vi "PC104_interface_GUI.vi"(8 "error in (no error)":errorcluster, 9 "URL prefex":string, 10 "Http session":T1, 11 "go":bool=TRUE) -> (2 "error out":errorcluster, 3 "Cluster":T2)   [LabVIEW 2017]
uses:
  Type_Defs/Digital_Out.ctl
  Type_Defs/Digital_In_1.ctl
  Type_Defs/Digital_In_SW_Wire_Faults.ctl
  Type_Defs/Digital_In_SW_States.ctl
  <vilib>/httpClient/ClientHandle.ctl
  msg7171_linux.llb/send single message.vi
  msg7171_linux.llb/send multiple messages.vi
  <vilib>/httpClient/POSTBuffer.vi
  <vilib>/httpClient/LabVIEWHTTPClient.lvlib
panel:
  out "Digi_In_SW_status":T3
  out "Digi_In_SW: Wire Faults":T4
  out "GetAIO json":string
  out "GetDIO json":string
  in  "Get AIO":bool=TRUE
  in  "IR Lamps DutyCycle":dbl[][](array[numeric]) format="%#.4g"
  in  "LN2 Platen":u16(slide) max=2047 step=1 scale=0.0..2047.0
  in  "LN2 Shroud":u16(slide) max=2047 step=1 scale=0.0..2047.0
  out "Digi_In_Bits":T5
  in  "Digi_Out":T6
  in  "Get DIO":bool=TRUE
  in  "exit":bool
  # "1"
  # "15"
  # "2"
  # "16"
  # "2              4              6              8              10            12            14          16"
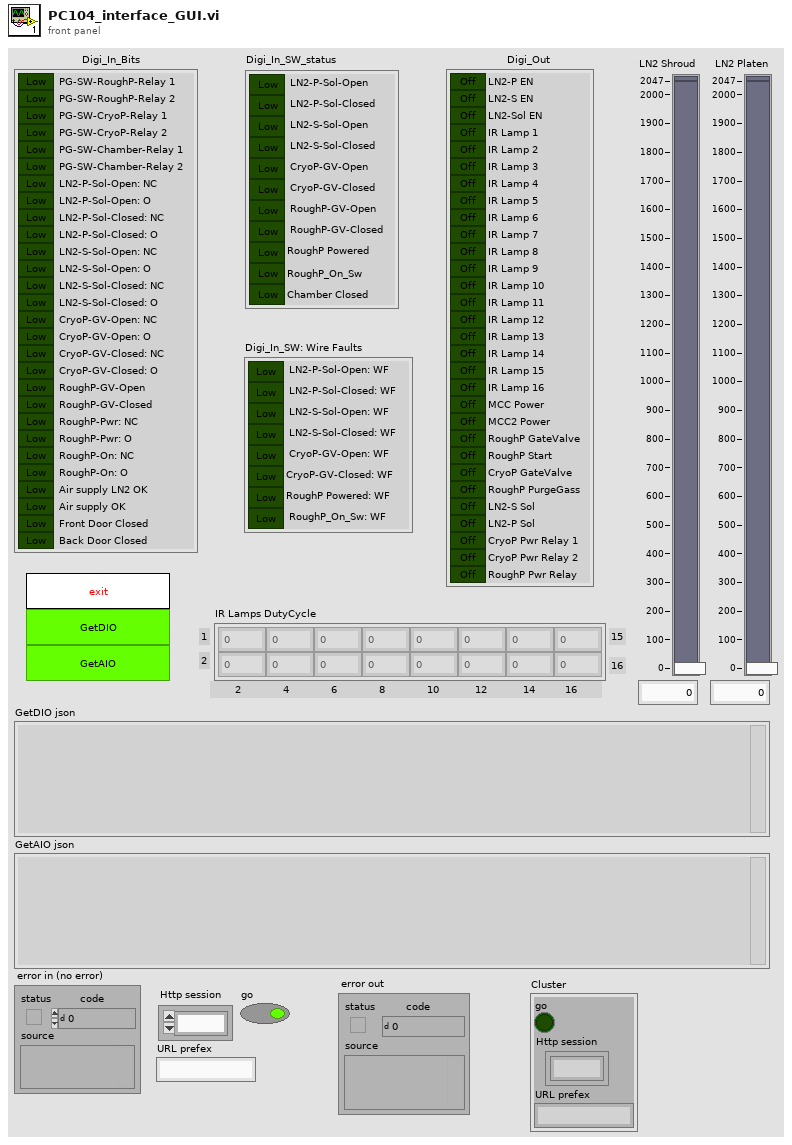
[diagram p1: front panel]
types:
  T1 = typedef "LabVIEWHTTPClient.lvlib/ClientHandle.ctl" = refnum<k1>
  T2 = cluster{"go":bool, "Http session":T1, "URL prefex":string}
  T3 = typedef "Digital_In_SW_States.ctl" = cluster{"LN2-P-Sol-Open":bool, "LN2-P-Sol-Closed":bool, "LN2-S-Sol-Open":bool, "LN2-S-Sol-Closed":bool, "CryoP-GV-Open":bool, "CryoP-GV-Closed":bool, "RoughP-GV-Open":bool, "RoughP-GV-Closed":bool, "RoughP Powered":bool, "RoughP_On_Sw":bool, "Chamber Closed":bool}
  T4 = typedef "Digital_In_SW_Wire_Faults.ctl" = cluster{"LN2-P-Sol-Open: WF":bool, "LN2-P-Sol-Closed: WF":bool, "LN2-S-Sol-Open: WF":bool, "LN2-S-Sol-Closed: WF":bool, "CryoP-GV-Open: WF":bool, "CryoP-GV-Closed: WF":bool, "RoughP Powered: WF":bool, "RoughP_On_Sw: WF":bool}
  T5 = typedef "Digital_In_1.ctl" = cluster{"PG-SW-RoughP-Relay 1":bool, "PG-SW-RoughP-Relay 2":bool, "PG-SW-CryoP-Relay 1":bool, "PG-SW-CryoP-Relay 2":bool, "PG-SW-Chamber-Relay 1":bool, "PG-SW-Chamber-Relay 2":bool, "LN2-P-Sol-Open: NC":bool, "LN2-P-Sol-Open: O":bool, "LN2-P-Sol-Closed: NC":bool, "LN2-P-Sol-Closed: O":bool, "LN2-S-Sol-Open: NC":bool, "LN2-S-Sol-Open: O":bool, "LN2-S-Sol-Closed: NC":bool, "LN2-S-Sol-Closed: O":bool, "CryoP-GV-Open: NC":bool, "CryoP-GV-Open: O":bool, "CryoP-GV-Closed: NC":bool, "CryoP-GV-Closed: O":bool, "RoughP-GV-Open":bool, "RoughP-GV-Closed":bool, "RoughP-Pwr: NC":bool, "RoughP-Pwr: O":bool, "RoughP-On: NC":bool, "RoughP-On: O":bool, "Air supply LN2 OK":bool, "Air supply OK":bool, "Front Door Closed":bool, "Back Door Closed":bool}
  T6 = typedef "Digital_Out.ctl" = cluster{"LN2-P EN":bool, "LN2-S EN":bool, "LN2-Sol EN":bool, "IR Lamp 1":bool, "IR Lamp 2":bool, "IR Lamp 3":bool, "IR Lamp 4":bool, "IR Lamp 5":bool, "IR Lamp 6":bool, "IR Lamp 7":bool, "IR Lamp 8":bool, "IR Lamp 9":bool, "IR Lamp 10":bool, "IR Lamp 11":bool, "IR Lamp 12":bool, "IR Lamp 13":bool, "IR Lamp 14":bool, "IR Lamp 15":bool, "IR Lamp 16":bool, "MCC Power":bool, "MCC2 Power":bool, "RoughP GateValve":bool, "RoughP Start":bool, "CryoP GateValve":bool, "RoughP PurgeGass":bool, "LN2-S Sol":bool, "LN2-P Sol":bool, "CryoP Pwr Relay 1":bool, "CryoP Pwr Relay 2":bool, "RoughP Pwr Relay":bool}
  T7 = cluster{"out":T6, "in bits":T5, "in sw":T3, "sw wf":T4}
  T8 = cluster{"out":cluster{"LN2 Platen":u16, "LN2 Shroud":u16}}
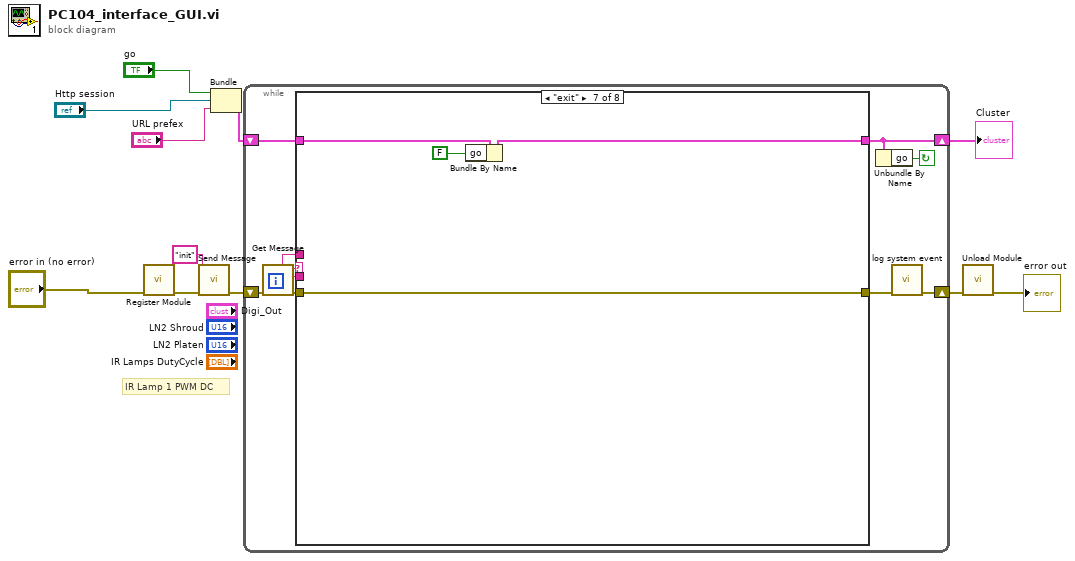
[diagram p0: block diagram]
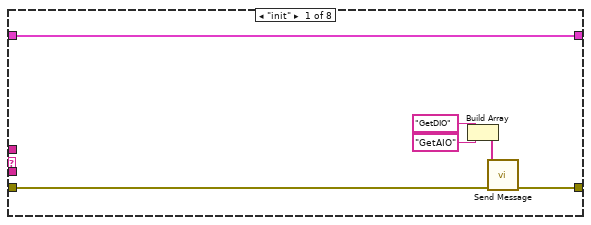
[diagram p2: hidden frame]
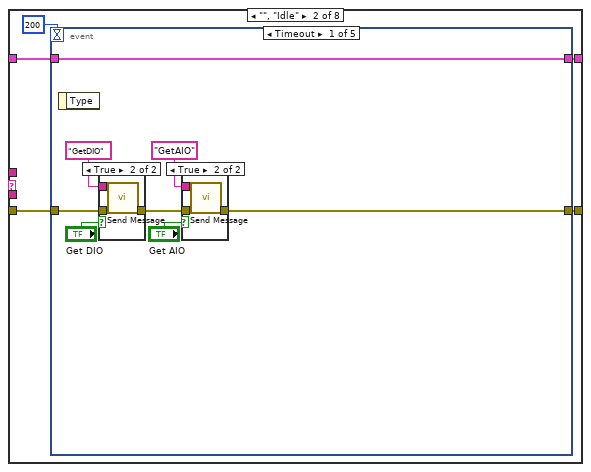
[diagram p3: hidden frame]
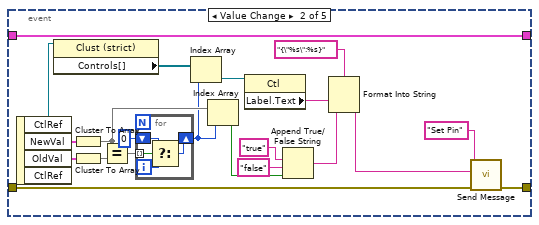
[diagram p6: hidden frame]
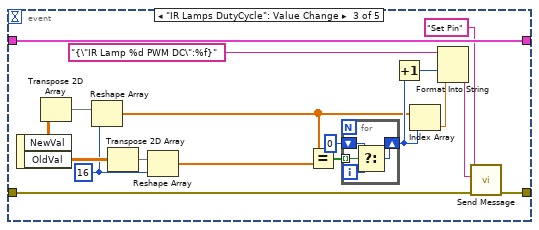
[diagram p7: hidden frame]
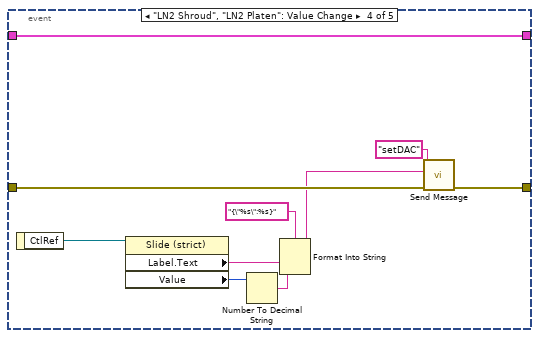
[diagram p8: hidden frame]
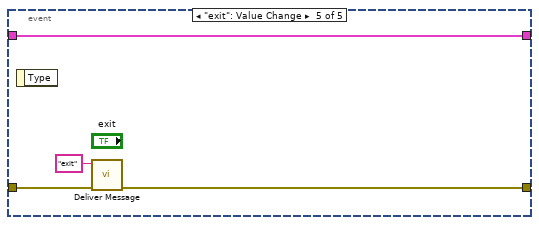
[diagram p9: hidden frame]
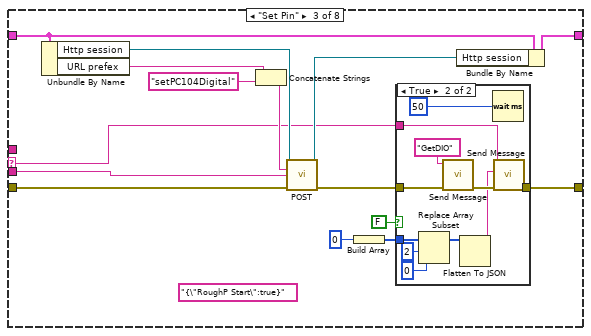
[diagram p10: hidden frame]
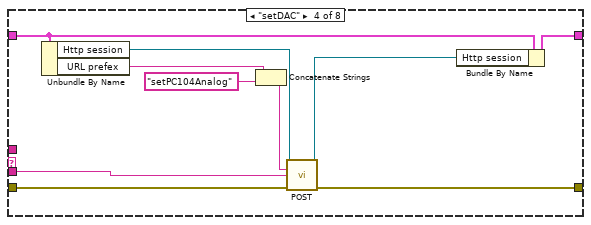
[diagram p12: hidden frame]
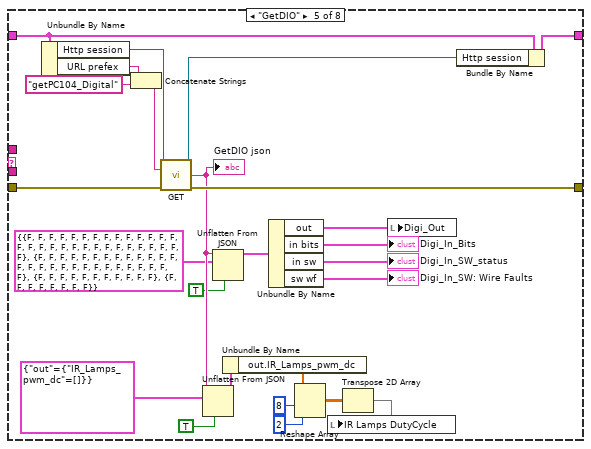
[diagram p13: hidden frame]
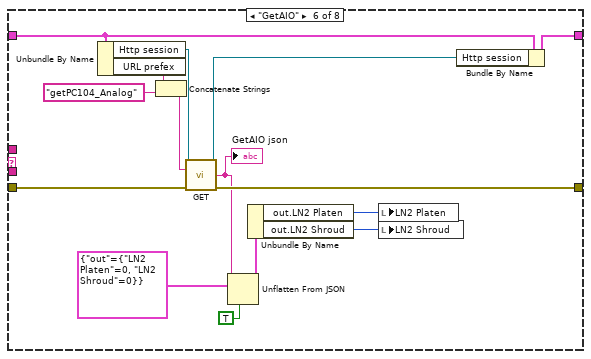
[diagram p14: hidden frame]
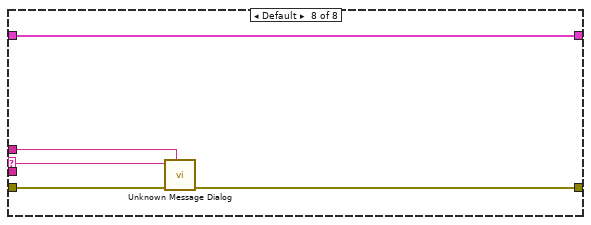
[diagram p15: hidden frame]
diagram:
  # "IR Lamp 1 PWM DC"
  n1 = call "Register Module.vi"("error in (no error)"="error in (no error)") -> ("error out"=w6:errorcluster)  [unwired: 9 in, 1 out]
  n2 = call-poly "Send Message.vi"("error in (no error)"=w6, "event"="init") -> ("error out"=w5:errorcluster)  [unwired: 9 in]
  n3 = Bundle("go"="go", "Http session"="Http session", "URL prefex"="URL prefex") -> (w11:T2)  [unwired: 1 in]
  n4 = while {
    shift-left: w11 -> [w18]
    shift-right: [w15] -> w1
    shift-right: [w13] -> w10
    shift-left: w5 -> [w21]
    stop <- w14 continue-if-true
    n5 = call "Get Message.vi"("error in (no error)"=w21) -> ("error out"=w19:errorcluster, "event buffer"=w20:string, "event"=w17:string, "source"=w16:string)  [unwired: 7 in]
    n6 = case shown="\"exit\"" w17 {
      selector: w17 -> [_ _ w115 _ _ _ _ w193]
      tunnel: [w23 w29 w119 w141 w164 w179 w190 w195] -> w15
      tunnel: w18 -> [w23 w28 w118 w140 w163 w178 w188 w195]
      tunnel: w20 -> [_ _ w113 w137 _ _ _ _]
      tunnel: w19 -> [w22 w30 w117 w139 w166 w181 w187 w194]
      tunnel: w16 -> [_ _ _ _ _ _ _ w192]
      tunnel: [w27 w32 w116 w138 w165 w180 w187 w191] -> w12
      frame "init" {
        n7 = Build Array("GetDIO" ("event"), "GetAIO" ("event")) -> (w25:string[])
        n8 = call-poly "Send Message.vi"("error in (no error)"=w22, "event"=w25) -> ("error out"=w27:errorcluster)  [unwired: 9 in]
      }
      frame "", "Idle" {
        n9 = event shown="[0] Timeout" {
          selector: _ -> [_ _ _ _ _]
          dyn-events: _ -> [_ _ _ _ _]
          timeout: 200 ("milliseconds to wait") -> [_ _ _ _ _]
          tunnel: w30 -> [w39 w64 w88 w103 w109]
          tunnel: [w34 w63 w87 w104 w108] -> w32
          tunnel: [w40 w69 w91 w96 w106] -> w29
          tunnel: w28 -> [w40 w69 w91 w96 w106]
          event Timeout {
            n10 = event-data() -> ()  [unwired: 1 in, 1 out]
            n11 = case shown="True" "Get DIO" {
              tunnel: w39 -> [w45 w48]
              tunnel: [w45 w47] -> w37
              tunnel: "GetDIO" ("event") -> [_ w46]
              frame False {
              }
              frame True {
                n12 = call-poly "Send Message.vi"("error in (no error)"=w48, "event"=w46) -> ("error out"=w47:errorcluster)  [unwired: 9 in]
              }
            }
            n13 = case shown="True" "Get AIO" {
              tunnel: w37 -> [w41 w44]
              tunnel: [w41 w43] -> w34
              tunnel: "GetAIO" ("event") -> [_ w42]
              frame False {
              }
              frame True {
                n14 = call-poly "Send Message.vi"("error in (no error)"=w44, "event"=w42) -> ("error out"=w43:errorcluster)  [unwired: 9 in]
              }
            }
          }
          event Value Change {
            n15 = event-data() -> ("CtlRef"=w50:refnum<vi>, "NewVal"=w65:T6, "OldVal"=w68:T6)  [unwired: 1 in, 1 out]
            n16 = property class="Clust (strict)"(reference=w50) -> ("Controls[]"=w60:refnum<vi>[])  [unwired: 1 in, 2 out]
            n17 = Cluster To Array(cluster=w65) -> (array=w61:bool[])
            n18 = Cluster To Array(cluster=w68) -> (array=w62:bool[])
            n19 = Equal?(x=w61, y=w62) -> (x = y?=w67:bool[])
            n20 = for {
              tunnel: w67 -> [w73] mode=indexing
              shift-right: [w72] -> w59
              shift-left: 0 -> [w71]
              i -> [w70]
              n21 = Select(t=w71, s=w73, f=w70) -> (s? t:f=w72:i32)
            }
            n22 = Index Array(array=w60, index=w59) -> (element=w58:refnum<vi>)
            n23 = Index Array(array=w61, index=w59) -> (element=w56:bool)
            n24 = property class="Ctl"(reference=w58) -> ("Label.Text"=w53:string)  [unwired: 1 in, 2 out]
            n25 = Append True/False String(1:w56, 2:"false" ("false string"), 3:"true" ("true string")) -> (0:w51:string)  [unwired: 1 in]
            n26 = Format Into String(format string="{\"%s\":%s}" ("string"), w53, w51) -> (resulting string=w49:string)  [unwired: 2 in, 1 out]
            n27 = call-poly "Send Message.vi"("error in (no error)"=w64, "event buffer"=w49, "event"="Set Pin") -> ("error out"=w63:errorcluster)  [unwired: 8 in]
          }
          event "IR Lamps DutyCycle": Value Change {
            w76 = 16 ("dimension size")
            n28 = event-data() -> ("NewVal"=w81:dbl[][], "OldVal"=w78:dbl[][])  [unwired: 1 in]
            n29 = Transpose 2D Array(2D array=w81) -> (transposed array=w82:dbl[][])
            n30 = Reshape Array(w82, w76) -> (w80:dbl[])
            n31 = Transpose 2D Array(2D array=w78) -> (transposed array=w79:dbl[][])
            n32 = Reshape Array(w79, w76) -> (w77:dbl[])
            n33 = Equal?(x=w80, y=w77) -> (x = y?=w90:bool[])
            n34 = for {
              tunnel: w90 -> [w95] mode=indexing
              shift-right: [w94] -> w83
              shift-left: 0 -> [w93]
              i -> [w92]
              n35 = Select(t=w93, s=w95, f=w92) -> (s? t:f=w94:i32)
            }
            n36 = Increment(x=w83) -> (x+1=w74:i32)
            n37 = Index Array(array=w80, index=w83) -> (element=w75:dbl)
            n38 = Format Into String(format string="{\"IR Lamp %d PWM DC\":%f}" ("string"), w74, w75) -> (resulting string=w84:string)  [unwired: 2 in, 1 out]
            n39 = call-poly "Send Message.vi"("error in (no error)"=w88, "event buffer"=w84, "event"="Set Pin") -> ("error out"=w87:errorcluster)  [unwired: 8 in]
          }
          event "LN2 Shroud", "LN2 Platen": Value Change {
            n40 = event-data() -> ("CtlRef"=w102:refnum<vi>)  [unwired: 1 in]
            n41 = property class="Slide (strict)"(reference=w102) -> ("Label.Text"=w100:string, "Value"=w99:u16)  [unwired: 1 in, 2 out]
            n42 = Number To Decimal String(number=w99) -> (decimal integer string=w98:string)  [unwired: 1 in]
            n43 = Format Into String(format string="{\"%s\":%s}" ("string"), w100, w98) -> (resulting string=w97:string)  [unwired: 2 in, 1 out]
            n44 = call-poly "Send Message.vi"("error in (no error)"=w103, "event buffer"=w97, "event"="setDAC") -> ("error out"=w104:errorcluster)  [unwired: 8 in]
          }
          event "exit": Value Change {
            n45 = event-data() -> ()  [unwired: 1 in, 1 out]
            n46 = call "Deliver Message.vi"("error in (no error)"=w109, "event"="exit") -> ("error out"=w108:errorcluster)  [unwired: 9 in]
          }
        }
      }
      frame "Set Pin" {
        (unwired) "{\"RoughP Start\":true}" ("string")
        n47 = Unbundle By Name(w118) -> ("Http session"=w123:T1, "URL prefex"=w121:string)
        n48 = Concatenate Strings(w121, "setPC104Digital" ("url")) -> (w122:string)
        n49 = call-poly <vilib>:"POST.vi"("client handle"=w123, "url"=w122, "buffer"=w113, "error in (no error)"=w117) -> ("client handle out"=w124:T1, "error out"=w114:errorcluster)  [unwired: 8 in, 2 out]
        n50 = Build Array(0) -> (w111:i32[])
        n51 = case shown="True" FALSE {
          tunnel: [w125 w136] -> w116
          tunnel: w115 -> [_ w135]
          tunnel: w114 -> [w125 w134]
          tunnel: w111 -> [_ w131]
          frame False {
          }
          frame True {
            n52 = Replace Array Subset(array=w131, new element=0 ("new element/subarray"), index=2) -> (w127:i32[])
            n53 = call-poly "Send Message.vi"("error in (no error)"=w134, "event"="GetDIO") -> ("error out"=w133:errorcluster)  [unwired: 9 in]
            n54 = Flatten To JSON(anything=w127) -> (JSON string=w128:string)  [unwired: 2 in, 1 out]
            n55 = Wait (ms)(milliseconds to wait=u32 50) -> ()  [unwired: 1 out]
            n56 = call-poly "Send Message.vi"("error in (no error)"=w133, "event buffer"=w128, "event"=w135) -> ("error out"=w136:errorcluster)  [unwired: 8 in]
          }
        }
        n57 = Bundle By Name(cluster=w118, "Http session"=w124) -> (w119:T2)
      }
      frame "setDAC" {
        n58 = Unbundle By Name(w140) -> ("Http session"=w145:T1, "URL prefex"=w143:string)
        n59 = Concatenate Strings(w143, "setPC104Analog" ("url")) -> (w144:string)
        n60 = call-poly <vilib>:"POST.vi"("client handle"=w145, "url"=w144, "buffer"=w137, "error in (no error)"=w139) -> ("client handle out"=w146:T1, "error out"=w138:errorcluster)  [unwired: 8 in, 2 out]
        n61 = Bundle By Name(cluster=w140, "Http session"=w146) -> (w141:T2)
      }
      frame "GetDIO" {
        n62 = Unbundle By Name(w163) -> ("Http session"=w170:T1, "URL prefex"=w168:string)
        n63 = Concatenate Strings(w168, "getPC104_Digital" ("url")) -> (w169:string)
        n64 = call <vilib>:"GET.vi"("client handle"=w170, "url"=w169, "error in (no error)"=w166) -> ("client handle out"=w171:T1, "body"=w152:string, "error out"=w165:errorcluster)  [unwired: 9 in, 1 out]
        "GetDIO json" <- w152
        n65 = Unflatten From JSON(JSON string=w152, type and defaults=cluster{"out":cluster{"IR_Lamps_pwm_dc":dbl[]}} {"out"={"IR_Lamps_pwm_dc"=[]}}, default null elements? (F)=TRUE) -> (value=w154:cluster{"out":cluster{"IR_Lamps_pwm_dc":dbl[]}})  [unwired: 4 in, 1 out]
        n66 = Unflatten From JSON(JSON string=w152, type and defaults=T7 {"out"={"LN2-P EN"=FALSE, "LN2-S EN"=FALSE, "LN2-Sol EN"=FALSE, "IR Lamp 1"=FALSE, "IR Lamp 2"=FALSE, "IR Lamp 3"=FALSE, "IR Lamp 4"=FALSE, "IR Lamp 5"=FALSE, "IR Lamp 6"=FALSE, "IR Lamp 7"=FALSE, "IR Lamp 8"=FALSE, "IR Lamp 9"=FALSE, "IR Lamp 10"=FALSE, "IR Lamp 11"=FALSE, "IR Lamp 12"=FALSE, "IR Lamp 13"=FALSE, "IR Lamp 14"=FALSE, "IR Lamp 15"=FALSE, "IR Lamp 16"=FALSE, "MCC Power"=FALSE, "MCC2 Power"=FALSE, "RoughP GateValve"=FALSE, "RoughP Start"=FALSE, "CryoP GateValve"=FALSE, "RoughP PurgeGass"=FALSE, "LN2-S Sol"=FALSE, "LN2-P Sol"=FALSE, "CryoP Pwr Relay 1"=FALSE, "CryoP Pwr Relay 2"=FALSE, "RoughP Pwr Relay"=FALSE}, "in bits"={"PG-SW-RoughP-Relay 1"=FALSE, "PG-SW-RoughP-Relay 2"=FALSE, "PG-SW-CryoP-Relay 1"=FALSE, "PG-SW-CryoP-Relay 2"=FALSE, "PG-SW-Chamber-Relay 1"=FALSE, "PG-SW-Chamber-Relay 2"=FALSE, "LN2-P-Sol-Open: NC"=FALSE, "LN2-P-Sol-Open: O"=FALSE, "LN2-P-Sol-Closed: NC"=FALSE, "LN2-P-Sol-Closed: O"=FALSE, "LN2-S-Sol-Open: NC"=FALSE, "LN2-S-Sol-Open: O"=FALSE, "LN2-S-Sol-Closed: NC"=FALSE, "LN2-S-Sol-Closed: O"=FALSE, "CryoP-GV-Open: NC"=FALSE, "CryoP-GV-Open: O"=FALSE, "CryoP-GV-Closed: NC"=FALSE, "CryoP-GV-Closed: O"=FALSE, "RoughP-GV-Open"=FALSE, "RoughP-GV-Closed"=FALSE, "RoughP-Pwr: NC"=FALSE, "RoughP-Pwr: O"=FALSE, "RoughP-On: NC"=FALSE, "RoughP-On: O"=FALSE, "Air supply LN2 OK"=FALSE, "Air supply OK"=FALSE, "Front Door Closed"=FALSE, "Back Door Closed"=FALSE}, "in sw"={"LN2-P-Sol-Open"=FALSE, "LN2-P-Sol-Closed"=FALSE, "LN2-S-Sol-Open"=FALSE, "LN2-S-Sol-Closed"=FALSE, "CryoP-GV-Open"=FALSE, "CryoP-GV-Closed"=FALSE, "RoughP-GV-Open"=FALSE, "RoughP-GV-Closed"=FALSE, "RoughP Powered"=FALSE, "RoughP_On_Sw"=FALSE, "Chamber Closed"=FALSE}, "sw wf"={"LN2-P-Sol-Open: WF"=FALSE, "LN2-P-Sol-Closed: WF"=FALSE, "LN2-S-Sol-Open: WF"=FALSE, "LN2-S-Sol-Closed: WF"=FALSE, "CryoP-GV-Open: WF"=FALSE, "CryoP-GV-Closed: WF"=FALSE, "RoughP Powered: WF"=FALSE, "RoughP_On_Sw: WF"=FALSE}}, default null elements? (F)=TRUE) -> (value=w160:T7)  [unwired: 4 in, 1 out]
        n67 = Unbundle By Name(w154) -> ("out.IR_Lamps_pwm_dc"=w153:dbl[])
        n68 = Unbundle By Name(w160) -> ("out"=w162:T6, "in bits"=→"Digi_In_Bits":T5, "in sw"=→"Digi_In_SW_status":T3, "sw wf"=→"Digi_In_SW: Wire Faults":T4)
        n69 = Reshape Array(w153, 8 ("dimension size"), 2 ("dimension size")) -> (w157:dbl[][])
        n70 = Transpose 2D Array(2D array=w157) -> (transposed array=w156:dbl[][])
        n71 = local write "IR Lamps DutyCycle"(w156) -> ()
        n72 = local write "Digi_Out"(w162) -> ()
        n73 = Bundle By Name(cluster=w163, "Http session"=w171) -> (w164:T2)
      }
      frame "GetAIO" {
        n74 = Unbundle By Name(w178) -> ("Http session"=w185:T1, "URL prefex"=w183:string)
        n75 = Concatenate Strings(w183, "getPC104_Analog" ("url")) -> (w184:string)
        n76 = call <vilib>:"GET.vi"("client handle"=w185, "url"=w184, "error in (no error)"=w181) -> ("client handle out"=w186:T1, "body"=w173:string, "error out"=w180:errorcluster)  [unwired: 9 in, 1 out]
        "GetAIO json" <- w173
        n77 = Unflatten From JSON(JSON string=w173, type and defaults=T8 {"out"={"LN2 Platen"=0, "LN2 Shroud"=0}}, default null elements? (F)=TRUE) -> (value=w176:T8)  [unwired: 4 in, 1 out]
        n78 = Unbundle By Name(w176) -> ("out.LN2 Platen"=w175:u16, "out.LN2 Shroud"=w174:u16)
        n79 = local write "LN2 Platen"(w175) -> ()
        n80 = local write "LN2 Shroud"(w174) -> ()
        n81 = Bundle By Name(cluster=w178, "Http session"=w186) -> (w179:T2)
      }
      frame "exit" {
        n82 = Bundle By Name(cluster=w188, "go"=FALSE ("Bundle Element")) -> (w190:T2)
      }
      frame Default {
        n83 = call "Unknown Message Dialog.vi"("source"=w192, "error in (no error)"=w194, "event name"=w193) -> ("error out"=w191:errorcluster)  [unwired: 8 in]
      }
    }
    n84 = Unbundle By Name(w15) -> ("go"=w14:bool)
    n85 = call "log system event.vi"("error in (no error)"=w12) -> ("error out"=w13:errorcluster)  [unwired: 9 in, 1 out]
  }
  "Cluster" <- w1
  n86 = call "Unload Module.vi"("error in (no error)"=w10) -> ("error out"=→"error out":errorcluster)  [unwired: 10 in]
